vi "Edit_Channel_Panel.vi"(0 "All Channel names":string[](array[string])=["30-10-03:New:Channel new5"], 9 "Result files to read":path[](array[path])) -> (3 "New Values Out":string[](array[string])=["Test data5"], 4 "New Chs Out":string[](array[string])=["30-10-03:New:Channel new5"], 6 "Cancelled":bool, 8 "Edit Raw Data Header Info Out":bool, 10 "Plotted rows only?":bool, 12 "ptUnderCursor":bool, 13 "Edit Raw data files?":bool, 14 "Raw data files in Orig Positions?":bool, 15 "Mode":T1)   [LabVIEW 2020]
uses:
  Plotter_Mode.ctl
panel:
  in  "Select channel names":bool
  in  "Cancel":bool
  in  "Edit Raw data files":i32(listbox)=1
  in  "Columns to Output":i32[](listbox)
  in  "Edit Type":i32(listbox)
  in  "OK Button":bool
  in  "Add values to:":i32(listbox)=1
  in  "New Values In":string[](array[string])=["Value"]
  in  "New Chs In":string[](array[string])=["Channel Name"]
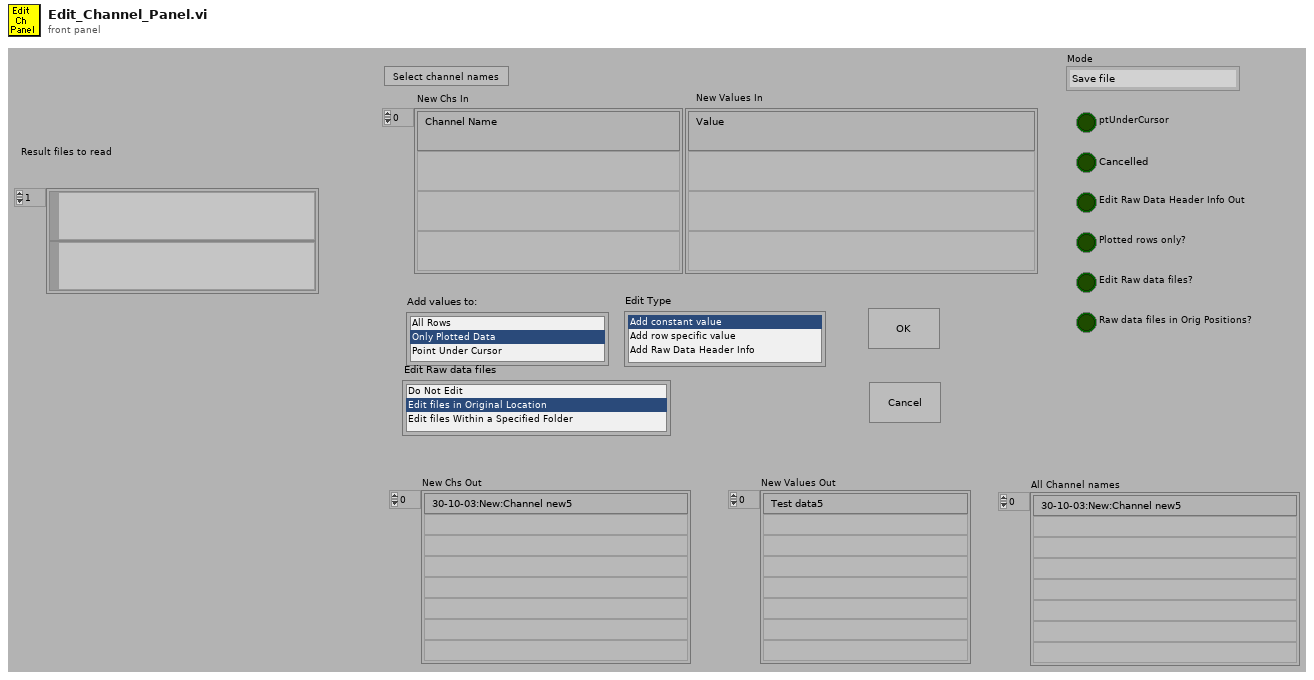
[diagram p1: front panel]
types:
  T1 = typedef "Plotter_Mode.ctl" = enum16{"Save file", "Delete unwanted rows", "Edit Values with constants", "Edit values per row", "Edit Raw Data file header", "Post Process Plotted Rows", "Plot EnFlo Tunnel Display", "Add Inlet Temperature Offset"}
  T2 = enum16{"Read Channels From File", "Read Channels from Server"}
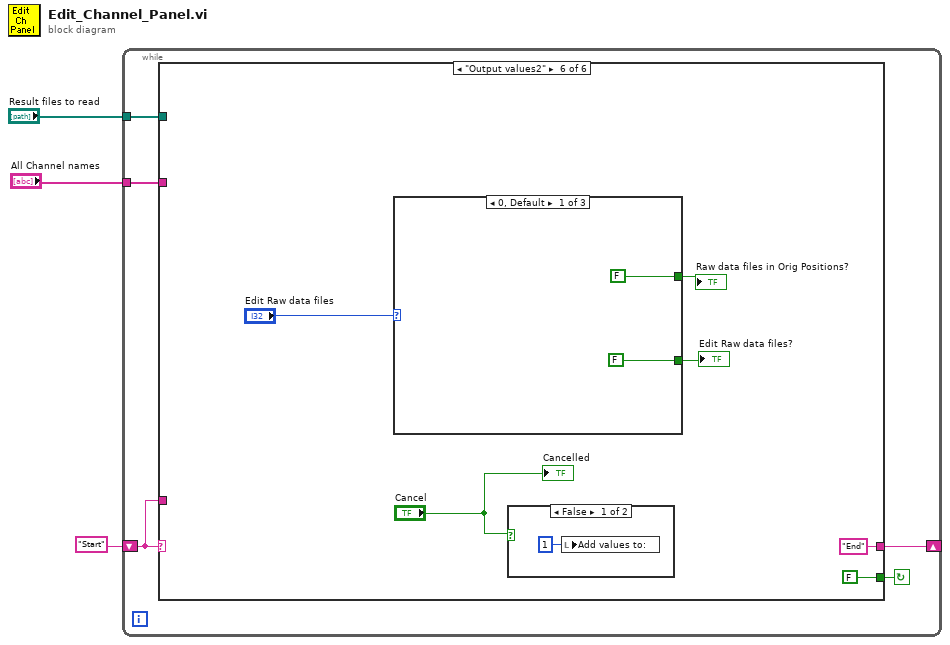
[diagram p0: block diagram]
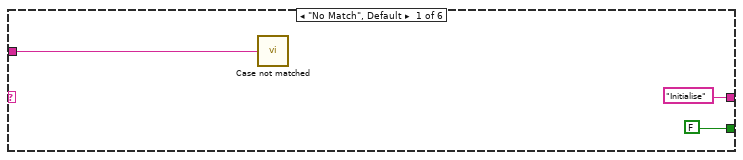
[diagram p2: hidden frame]
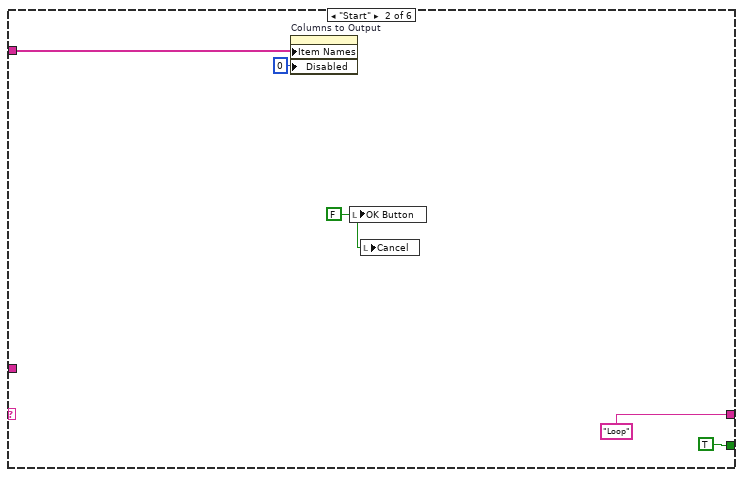
[diagram p3: hidden frame]
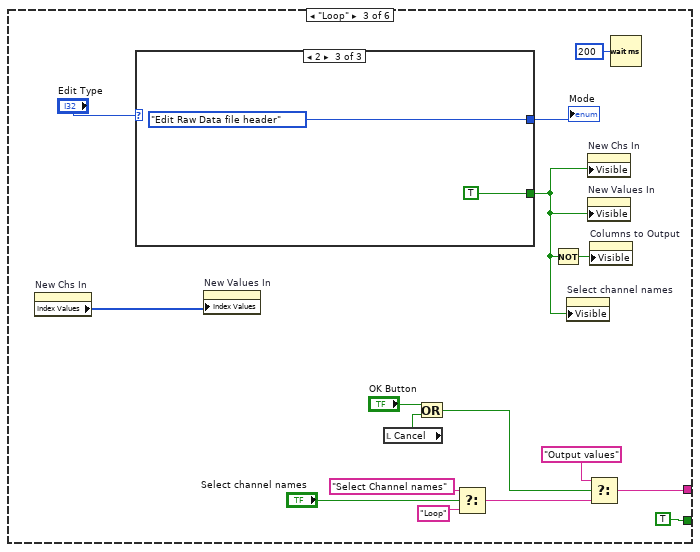
[diagram p4: hidden frame]
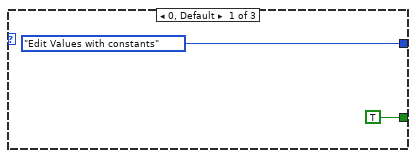
[diagram p5: hidden frame]
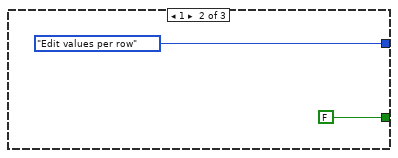
[diagram p6: hidden frame]
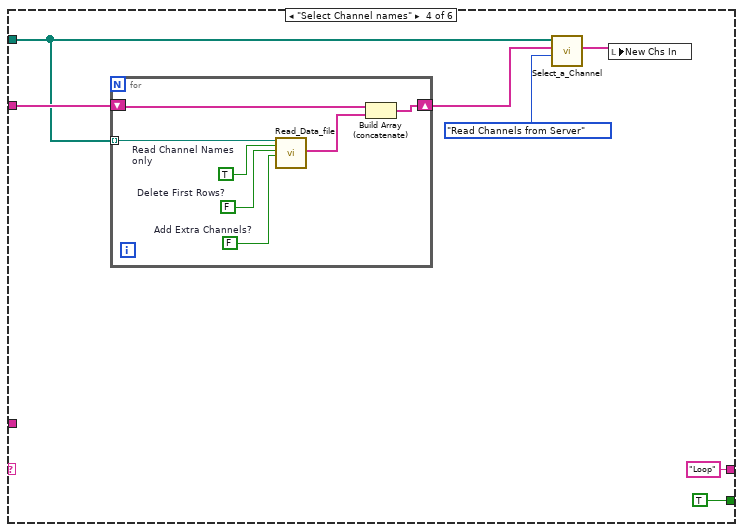
[diagram p7: hidden frame]
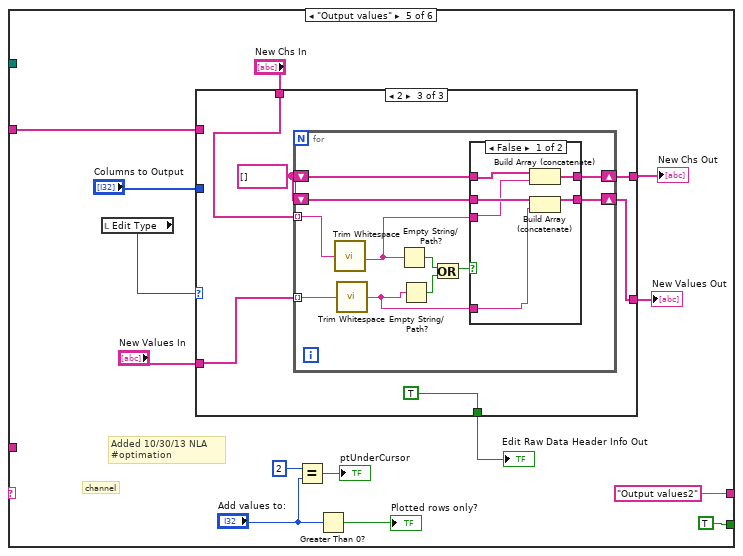
[diagram p8: hidden frame]
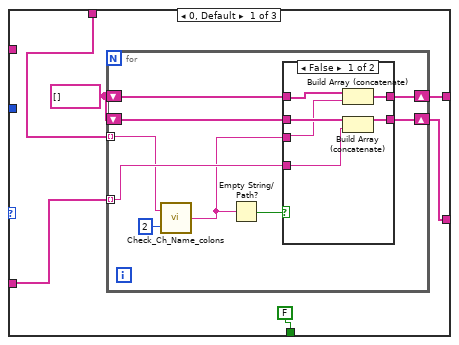
[diagram p9: hidden frame]
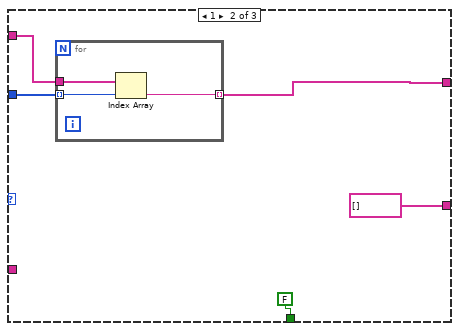
[diagram p11: hidden frame]
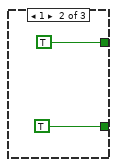
[diagram p14: hidden frame]
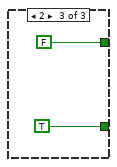
[diagram p15: hidden frame]
diagram:
  n1 = while {
    shift-left: "Start" -> [w6]
    shift-right: [w7] -> _
    tunnel: "All Channel names" -> [w5]
    tunnel: "Result files to read" -> [w4]
    stop <- w8 continue-if-true
    n2 = case shown="\"Output values2\"" w6 {
      tunnel: [FALSE TRUE TRUE TRUE TRUE FALSE] -> w8
      tunnel: ["Initialise" "Loop" w30 "Loop" "Output values2" "End"] -> w7
      tunnel: w6 -> [w9 _ _ _ _ _]
      tunnel: w5 -> [_ w14 _ w44 w57 _]
      tunnel: w4 -> [_ _ _ w39 _ _]
      frame "No Match", Default {
        n3 = call "Case not matched.vi"("Case Name not Matched"=w9) -> ()
      }
      frame "Start" {
        w12 = FALSE ("OK Button")
        n4 = property on="Columns to Output" class="LstBox (strict)"("Item Names"=w14, "Disabled"=u8 0) -> ()  [unwired: 2 in, 2 out]
        n5 = local write "OK Button"(w12) -> ()
        n6 = local write "Cancel"(w12) -> ()
      }
      frame "Loop" {
        n7 = property on="New Chs In" class="Arr (strict)"() -> ("Index Values"=w20:u32[])  [unwired: 2 in, 2 out]
        n8 = case shown="2" "Edit Type" {
          tunnel: [Plotter_Mode."Edit Values with constants" ("Mode") Plotter_Mode."Edit values per row" ("Mode") Plotter_Mode."Edit Raw Data file header" ("Mode")] -> w28
          tunnel: [TRUE FALSE TRUE] -> w17
          frame 0, Default {
          }
          frame 1 {
          }
          frame 2 {
          }
        }
        "Mode" <- w28
        n9 = property on="New Values In" class="Arr (strict)"("Index Values"=w20) -> ()  [unwired: 2 in, 2 out]
        n10 = local read "Cancel"() -> (w26:bool)
        n11 = Or(x="OK Button", y=w26) -> (x .or. y?=w24:bool)
        n12 = Select(t="Select Channel names", s="Select channel names", f="Loop") -> (s? t:f=w19:string)
        n13 = Not(x=w17) -> (.not. x?=w27:bool)
        n14 = property on="Select channel names" class="Bool"("Visible"=w17) -> ()  [unwired: 2 in, 2 out]
        n15 = property on="New Chs In" class="Arr (strict)"("Visible"=w17) -> ()  [unwired: 2 in, 2 out]
        n16 = property on="New Values In" class="Arr (strict)"("Visible"=w17) -> ()  [unwired: 2 in, 2 out]
        n17 = Select(t="Output values", s=w24, f=w19) -> (s? t:f=w30:string)
        n18 = property on="Columns to Output" class="LstBox (strict)"("Visible"=w27) -> ()  [unwired: 2 in, 2 out]
        n19 = Wait (ms)(milliseconds to wait=u32 200) -> ()  [unwired: 1 out]
      }
      frame "Select Channel names" {
        n20 = for {
          shift-right: [w50] -> w43
          shift-left: w44 -> [w48]
          tunnel: w39 -> [w52] mode=indexing
          w46 = FALSE  # Delete First Rows?
          w47 = FALSE  # Add Extra Channels?
          w51 = TRUE  # Read Channel Names only
          n21 = call "Read_Data_file.vi"("Results file"=w52, "Read Channel Names only"=w51, "Delete First Rows?"=w46, "Add Extra Channels?"=w47) -> ("Ch names Out"=w49:string[])  [unwired: 3 in, 12 out]
          n22 = Build Array (concatenate)(w48, w49) -> (w50:string[])
        }
        n23 = call "Select_a_Channel.vi"("Mode"=T2."Read Channels from Server", "Extra channel names"=w43, "Data Files"=w39) -> ("Selected Channel Names"=w42:string[])  [unwired: 5 out]
        n24 = local write "New Chs In"(w42) -> ()
      }
      frame "Output values" {
        # "Added 10/30/13 NLA\n#optimation"
        # "channel"
        n25 = local read "Edit Type"() -> (w63:i32)
        n26 = case shown="2" w63 {
          tunnel: "New Values In" -> [w70 _ w101]
          tunnel: [w69 string[] [] w100] -> w61
          tunnel: "New Chs In" -> [w71 _ w102]
          tunnel: [w68 w92 w99] -> w59
          tunnel: "Columns to Output" -> [_ w94 _]
          tunnel: w57 -> [_ w93 _]
          tunnel: [FALSE FALSE TRUE] -> w56
          frame 0, Default {
            w72 = string[] []
            n27 = for {
              tunnel: w70 -> [w77] mode=indexing
              shift-right: [w78] -> w68
              shift-left: w72 -> [w81]
              shift-right: [w80] -> w69
              shift-left: w72 -> [w79]
              tunnel: w71 -> [w76] mode=indexing
              n28 = call "Check_Ch_Name_colons.vi"("No of Colons"=2, "Ch Name in"=w76) -> ("Ch Name out"=w75:string)
              n29 = Empty String/Path?(string/path=w75) -> (empty?=w74:bool)
              n30 = case shown="False" w74 {
                tunnel: [w84 w89] -> w78
                tunnel: w81 -> [w87 w89]
                tunnel: [w85 w88] -> w80
                tunnel: w79 -> [w86 w88]
                tunnel: w77 -> [w82 _]
                tunnel: w75 -> [w83 _]
                frame False {
                  n31 = Build Array (concatenate)(w87, w83) -> (w84:string[])
                  n32 = Build Array (concatenate)(w86, w82) -> (w85:string[])
                }
                frame True {
                }
              }
            }
          }
          frame 1 {
            n33 = for {
              tunnel: w94 -> [w97] mode=indexing
              tunnel: w93 -> [w96]
              tunnel: [w95] -> w92 mode=indexing
              n34 = Index Array(array=w96, index=w97) -> (element=w95:string)
            }
          }
          frame 2 {
            w103 = string[] []
            n35 = for {
              tunnel: w101 -> [w109] mode=indexing
              shift-right: [w111] -> w99
              shift-left: w103 -> [w114]
              shift-right: [w113] -> w100
              shift-left: w103 -> [w112]
              tunnel: w102 -> [w110] mode=indexing
              n36 = call <vilib>:"Trim Whitespace.vi"("string"=w110) -> ("trimmed string"=w105:string)  [unwired: 1 in]
              n37 = call <vilib>:"Trim Whitespace.vi"("string"=w109) -> ("trimmed string"=w104:string)  [unwired: 1 in]
              n38 = Empty String/Path?(string/path=w105) -> (empty?=w107:bool)
              n39 = Empty String/Path?(string/path=w104) -> (empty?=w108:bool)
              n40 = Or(x=w107, y=w108) -> (x .or. y?=w106:bool)
              n41 = case shown="False" w106 {
                tunnel: [w117 w122] -> w111
                tunnel: w114 -> [w120 w122]
                tunnel: [w118 w121] -> w113
                tunnel: w112 -> [w119 w121]
                tunnel: w105 -> [w116 _]
                tunnel: w104 -> [w115 _]
                frame False {
                  n42 = Build Array (concatenate)(w120, w116) -> (w117:string[])
                  n43 = Build Array (concatenate)(w119, w115) -> (w118:string[])
                }
                frame True {
                }
              }
            }
          }
        }
        "New Values Out" <- w61
        "New Chs Out" <- w59
        "Edit Raw Data Header Info Out" <- w56
        n44 = Equal?(x=2, y="Add values to:") -> (x = y?=→"ptUnderCursor":bool)
        n45 = Greater Than 0?(x="Add values to:") -> (x > 0?=→"Plotted rows only?":bool)
      }
      frame "Output values2" {
        n46 = case shown="0, Default" "Edit Raw data files" {
          tunnel: [FALSE TRUE TRUE] -> w125
          tunnel: [FALSE TRUE FALSE] -> w124
          frame 0, Default {
          }
          frame 1 {
          }
          frame 2 {
          }
        }
        "Edit Raw data files?" <- w125
        "Raw data files in Orig Positions?" <- w124
        n47 = case shown="False" "Cancel" {
          frame False {
            n48 = local write "Add values to:"(1 ("Add values to:")) -> ()
          }
          frame True {
          }
        }
        "Cancelled" <- "Cancel"
      }
    }
  }
